vi "SaveTestData.vi"(11 "Cluster":T1) -> (1 "Result":bool, 3 "output cluster":T1)   [LabVIEW 2013]
uses:
  Control/Buffer.vi
panel:
  out "output array 2":string[][](array[string])
  out "output array":string[][](array[string])
  out "TestData":string
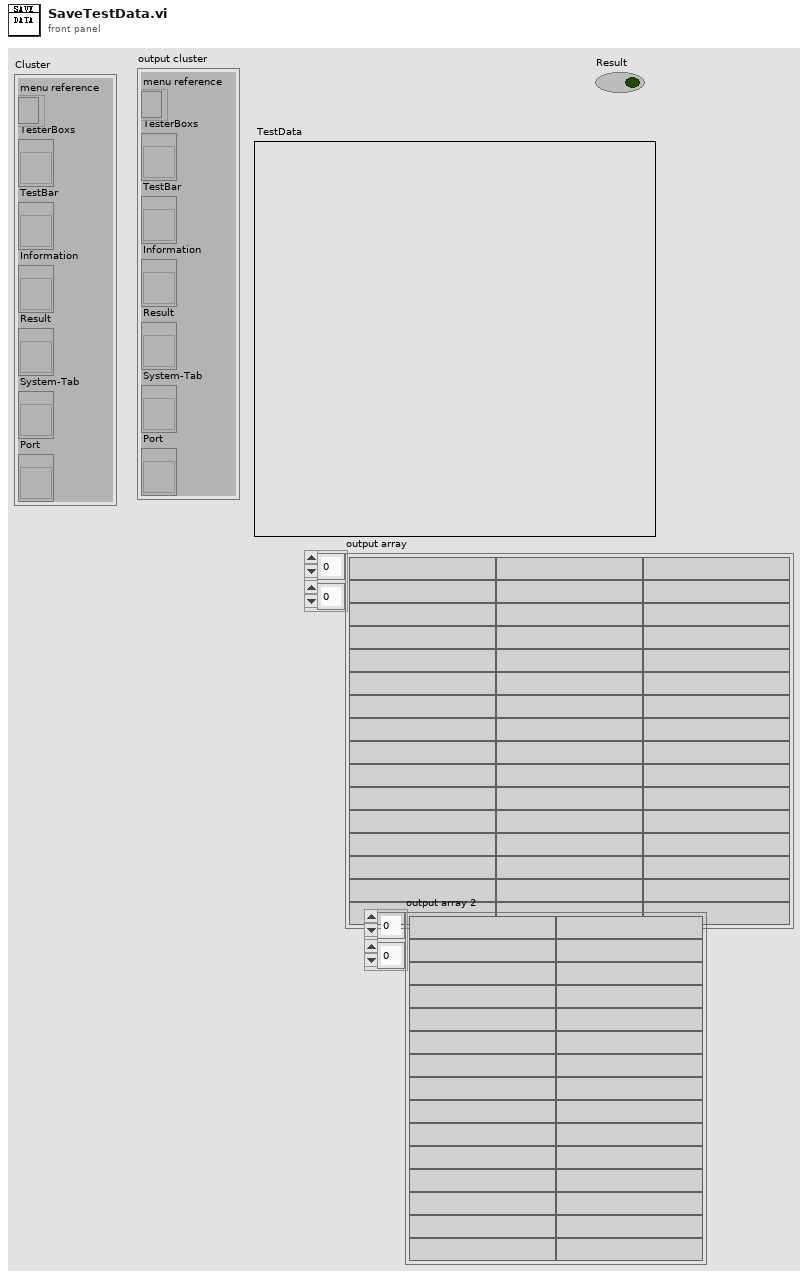
[diagram p1: front panel]
types:
  T1 = cluster{"menu reference":refnum<k9>, "TesterBoxs":refnum<vi>, "TestBar":refnum<vi>, "Information":refnum<vi>, "Result":refnum<vi>, "System-Tab":refnum<vi>, "Port":refnum<vi>}
  T2 = enum16{"open", "replace", "create", "open or create", "replace or create", "replace or create with confirmation"}
  T3 = typedef "StatusInformation.ctl" = cluster{"FileName:":string, "Barcode(S/N):":string, "TestStep:":string, "TestTime:":string, "Station:":string, "Model:":string, "Line:":string, "Status:":string, "Series:":string, "Reserve:":string}
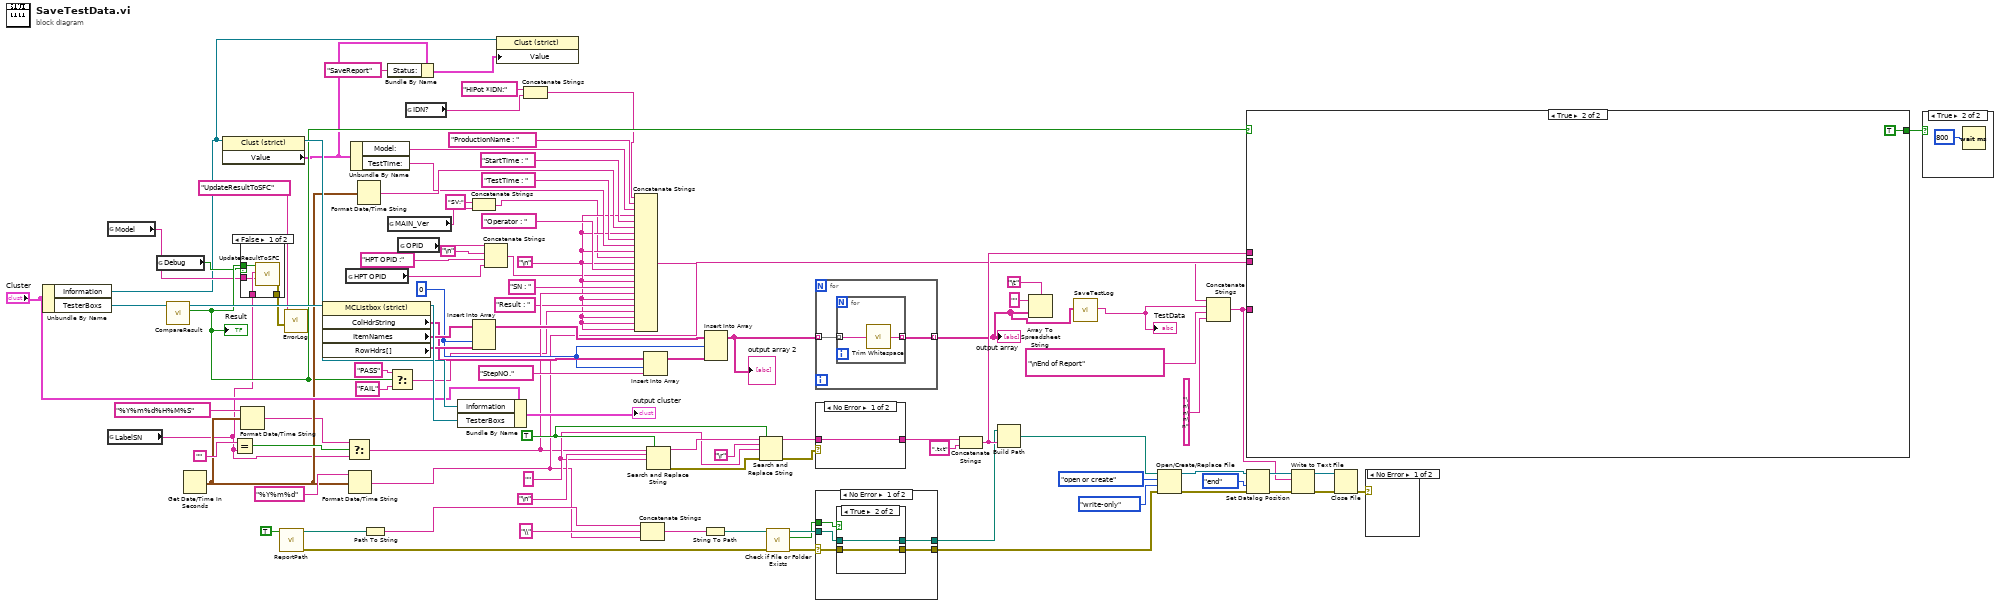
[diagram p0: block diagram]
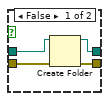
[diagram p3: hidden frame]
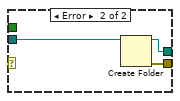
[diagram p4: hidden frame]
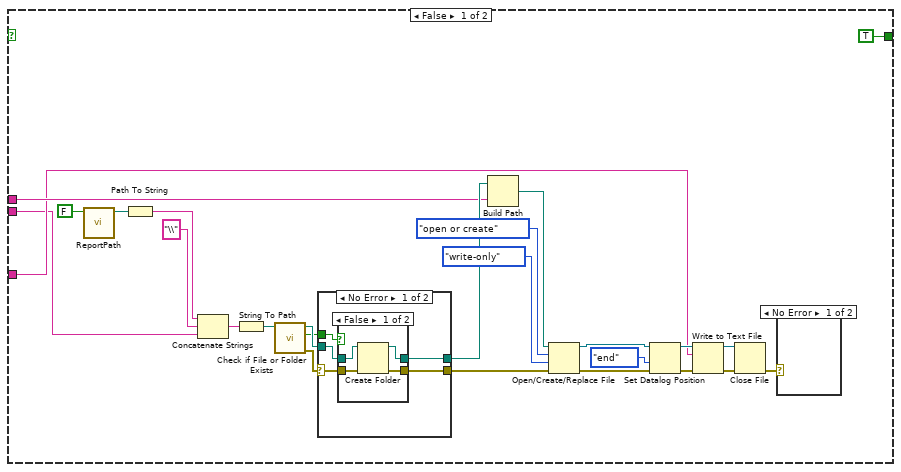
[diagram p6: hidden frame]
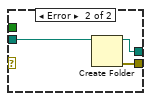
[diagram p9: hidden frame]
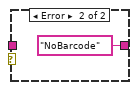
[diagram p11: hidden frame]
diagram:
  w91 = TRUE ("replace all? (F)")
  w89 = "" ("replace string (\"\")")
  w24 = "\n"
  w77 = 0 ("index (row)")
  n1 = Unbundle By Name("Cluster") -> ("Information"=w4:refnum<vi>, "TesterBoxs"=w76:refnum<vi>)
  n2 = global read "Buffer.vi" "Model"() -> (w11:string)
  n3 = global read "Buffer.vi" "LabelSN"() -> (w12:string)
  n4 = global read "Buffer.vi" "Debug"() -> (w8:bool)
  n5 = call "CompareResult.vi"("MulticolumnListbox in"=w76) -> ("Result"=w13:bool, "MulticolumnListbox out"=w75:refnum<vi>)  [unwired: 9 in]
  "Result" <- w13
  n6 = Get Date/Time In Seconds() -> (seconds since 1Jan1904=w41:timestamp)
  n7 = property class="Clust (strict)"(reference=w4) -> (reference out=w98:refnum<vi>, "Value"=w3:T3)  [unwired: 1 in, 1 out]
  n8 = Equal?(x="", y=w12) -> (x = y?=w44:bool)
  n9 = case shown="False" w8 {
    tunnel: w13 -> [w103 _]
    tunnel: w12 -> [w102 _]
    tunnel: w11 -> [w101 _]
    tunnel: [w100 _] -> w10
    frame False {
      n10 = call "UpdateResultToSFC.vi"("Message"=w101, "SN"=w102, "result"=w103) -> ("error out"=w100:errorcluster)  [unwired: 8 in]
    }
    frame True {
    }
  }
  n11 = Format Date/Time String(time format string (%c)="%Y%m%d%H%M%S", seconds (now)=w41) -> (date/time string=w39:string)  [unwired: 1 out]
  n12 = call "ReportPath.vi"("s"=TRUE) -> ("error out"=w49:errorcluster, "created path"=w57:path)  [unwired: 9 in]
  n13 = call "ErrorLog.vi"("error in (no error)"=w10, "Step No."="UpdateResultToSFC") -> ()  [unwired: 9 in, 1 out]
  n14 = property class="MCListbox (strict)"(reference=w75) -> (reference out=w99:refnum<vi>, "ColHdrString"=w80:string[], "ItemNames"=w82:string[][], "RowHdrs[]"=w97:string[])  [unwired: 1 in, 1 out]
  n15 = global read "Buffer.vi" "HPT OPID"() -> (w14:string)
  n16 = Select(t=w39, s=w44, f=w12) -> (s? t:f=w27:string)
  n17 = Format Date/Time String(time format string (%c)="%Y%m%d" ("时间格式字符串(%c)"), seconds (now)=w41) -> (date/time string=w42:string)  [unwired: 1 out]
  n18 = Unbundle By Name(w3) -> ("Model:"=w34:string, "TestTime:"=w30:string)
  n19 = Format Date/Time String(seconds (now)=w41) -> (date/time string=w32:string)  [unwired: 2 in]
  n20 = Path To String(path=w57) -> (string=w55:string)
  n21 = global read "Buffer.vi" "MAIN_Ver"() -> (w21:string)
  n22 = Bundle By Name(cluster=w3, "Status:"="SaveReport") -> (w2:T3)
  n23 = Select(t="PASS", s=w13, f="FAIL") -> (s? t:f=w25:string)
  n24 = global read "Buffer.vi" "OPID"() -> (w17:string)
  n25 = global read "Buffer.vi" "IDN?"() -> (w5:string)
  n26 = Bundle By Name(cluster="Cluster", "Information"=w98, "TesterBoxs"=w99) -> (→"output cluster":T1)
  n27 = Concatenate Strings("SV:" ("string"), w21) -> (w20:string)
  n28 = Insert Into Array(array=w82, index (col)=w77, new element=w97) -> (w81:string[][])  [unwired: 1 in]
  n29 = Concatenate Strings(w17, "\n", "HPT OPID :" ("string"), w14) -> (w18:string)
  n30 = property class="Clust (strict)"(reference=w4, "Value"=w2) -> ()  [unwired: 1 in, 2 out]
  n31 = Concatenate Strings("HiPot *IDN:" ("string"), w5) -> (w7:string)
  n32 = Concatenate Strings(w7, "ProductionName : " ("element"), w34, w24, "StartTime : " ("element"), w32, w24, "TestTime : " ("element"), w30, w24, w20, w24, "Operator : " ("element"), w18, w24, "SN : " ("element"), w27, w24, "Result : " ("element"), w25, w24, w24, w24) -> (w36:string)
  n33 = Concatenate Strings(w55, "\\" ("string"), w42) -> (w54:string)
  n34 = Insert Into Array(array=w80, index=w77, new element="StepNO." ("new element/subarray")) -> (w79:string[])
  n35 = Search and Replace String(replace all?=w91, input string=w27, search string="\n", replace string=w89) -> (result string=w92:string, error out=w93:errorcluster)  [unwired: 4 in, 2 out]
  n36 = String To Path(string=w54) -> (path=w53:path)
  n37 = Insert Into Array(array=w81, index (row)=w77, new element=w79) -> (w37:string[][])  [unwired: 1 in]
  "output array 2" <- w37
  n38 = Search and Replace String(replace all?=w91, input string=w92, search string="\r", replace string=w89, error in=w93) -> (result string=w83:string, error out=w85:errorcluster)  [unwired: 3 in, 2 out]
  n39 = call <vilib>:"Check if File or Folder Exists.vi"("error in (no error)"=w49, "path"=w53) -> ("error out"=w50:errorcluster, "file or folder exists?"=w51:bool, "dup path"=w52:path)  [unwired: 7 in]
  n40 = for {
    tunnel: w37 -> [w104] mode=indexing
    tunnel: [w105] -> w23 mode=indexing
    n41 = for {
      tunnel: w104 -> [w107] mode=indexing
      tunnel: [w106] -> w105 mode=indexing
      n42 = call <vilib>:"Trim Whitespace.vi"("string"=w107) -> ("trimmed string"=w106:string)  [unwired: 1 in]
    }
  }
  "output array" <- w23
  n43 = case shown="No Error" w85 {
    tunnel: [w108 "NoBarcode" ("result string")] -> w84
    tunnel: w83 -> [w108 _]
    frame No Error {
    }
    frame Error {
    }
  }
  n44 = case shown="No Error" w50 {
    selector: w50 -> [w111 _]
    tunnel: w52 -> [w114 w123]
    tunnel: w51 -> [w113 _]
    tunnel: [w112 w122] -> w48
    tunnel: [w110 w121] -> w47
    frame No Error {
      n45 = case shown="True" w113 {
        tunnel: w114 -> [w118 w120]
        tunnel: [w117 w120] -> w112
        tunnel: w111 -> [w116 w119]
        tunnel: [w115 w119] -> w110
        frame False {
          n46 = Create Folder(path (use dialog)=w118, error in=w116) -> (created path=w117:path, error out=w115:errorcluster)  [unwired: 1 in, 1 out]
        }
        frame True {
        }
      }
    }
    frame Error {
      n47 = Create Folder(path (use dialog)=w123) -> (created path=w122:path, error out=w121:errorcluster)  [unwired: 2 in, 1 out]
    }
  }
  n48 = Concatenate Strings(w84, ".txt" ("string")) -> (w62:string)
  n49 = Build Path(base path=w48, name or relative path=w62) -> (appended path=w72:path)
  n50 = Array To Spreadsheet String(delimiter (Tab)="\t", array=w23, 3:"" ("format string")) -> ()  [unwired: 1 out]
  n51 = call "SaveTestLog.vi"("output array 3"=w23) -> ("String 2"=w22:string)  [unwired: 10 in]
  "TestData" <- w22
  n52 = Open/Create/Replace File(file path (use dialog)=w72, error in=w47, operation (0:open)=T2."open or create", access (0:read/write)=enum16{"read/write", "read-only", "write-only"}."write-only") -> (refnum out=w69:refnum<file>, error out=w67:errorcluster)  [unwired: 2 in, 1 out]
  n53 = Concatenate Strings(w36, w22, "\nEnd of Report" ("string"), "\n\n\n\n" ("string")) -> (w61:string)
  n54 = case shown="True" w13 {
    tunnel: w42 -> [w127 _]
    tunnel: w62 -> [w133 _]
    tunnel: w61 -> [w131 _]
    tunnel: [TRUE TRUE] -> w60
    frame False {
      n55 = call "ReportPath.vi"("s"=FALSE) -> ("created path"=w129:path)  [unwired: 9 in, 1 out]
      n56 = Path To String(path=w129) -> (string=w126:string)
      n57 = Concatenate Strings(w126, "\\" ("string"), w127) -> (w125:string)
      n58 = String To Path(string=w125) -> (path=w145:path)
      n59 = call <vilib>:"Check if File or Folder Exists.vi"("path"=w145) -> ("error out"=w143:errorcluster, "file or folder exists?"=w146:bool, "dup path"=w147:path)  [unwired: 8 in]
      n60 = case shown="No Error" w143 {
        selector: w143 -> [w151 _]
        tunnel: w147 -> [w154 w163]
        tunnel: w146 -> [w153 _]
        tunnel: [w152 w162] -> w144
        tunnel: [w150 w161] -> w135
        frame No Error {
          n61 = case shown="False" w153 {
            tunnel: w154 -> [w158 w160]
            tunnel: [w157 w160] -> w152
            tunnel: w151 -> [w156 w159]
            tunnel: [w155 w159] -> w150
            frame False {
              n62 = Create Folder(path (use dialog)=w158, error in=w156) -> (created path=w157:path, error out=w155:errorcluster)  [unwired: 1 in, 1 out]
            }
            frame True {
            }
          }
        }
        frame Error {
          n63 = Create Folder(path (use dialog)=w163) -> (created path=w162:path, error out=w161:errorcluster)  [unwired: 2 in, 1 out]
        }
      }
      n64 = Build Path(base path=w144, name or relative path=w133) -> (appended path=w142:path)
      n65 = Open/Create/Replace File(file path (use dialog)=w142, error in=w135, operation (0:open)=T2."open or create", access (0:read/write)=enum16{"read/write", "read-only", "write-only"}."write-only") -> (refnum out=w140:refnum<file>, error out=w138:errorcluster)  [unwired: 2 in, 1 out]
      n66 = Set Datalog Position(4:w138, 5:enum16{"start", "end", "current"}."end" ("from (0:start)"), 7:w140) -> (0:w136:errorcluster, 3:w139:refnum<file>)  [unwired: 1 in]
      n67 = Write to Text File(file (use dialog)=w139, text=w131, error in=w136) -> (refnum out=w149:refnum<file>, error out=w148:errorcluster)  [unwired: 1 in, 1 out]
      n68 = Close File(refnum=w149, error in=w148) -> (error out=w134:errorcluster)  [unwired: 1 out]
      n69 = case shown="No Error" w134 {
        frame No Error {
        }
        frame Error {
        }
      }
    }
    frame True {
    }
  }
  n70 = Set Datalog Position(4:w67, 5:enum16{"start", "end", "current"}."end" ("from (0:start)"), 7:w69) -> (0:w65:errorcluster, 3:w68:refnum<file>)  [unwired: 1 in]
  n71 = Write to Text File(file (use dialog)=w68, text=w61, error in=w65) -> (refnum out=w87:refnum<file>, error out=w86:errorcluster)  [unwired: 1 in, 1 out]
  n72 = Close File(refnum=w87, error in=w86) -> (error out=w63:errorcluster)  [unwired: 1 out]
  n73 = case shown="No Error" w63 {
    frame No Error {
    }
    frame Error {
    }
  }
  n74 = case shown="True" w60 {
    frame False {
    }
    frame True {
      n75 = Wait (ms)(milliseconds to wait=u32 800) -> ()  [unwired: 1 out]
    }
  }
